vi "DriveSingleton.vi"(9 "Get/Set":enum16{"Get", "Set"}(ring), 11 "DriveBase.lvclass":refnum<class "DriveBase.lvclass">) -> (3 "DriveBase.lvclass 2":refnum<class "DriveBase.lvclass">)   [LabVIEW 2016, in "DriveBase.lvclass"]
uses:
  DriveBase.lvclass
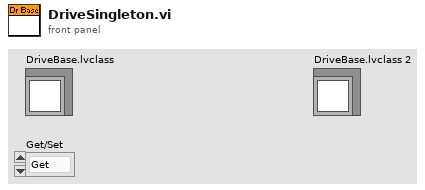
[diagram p1: front panel]
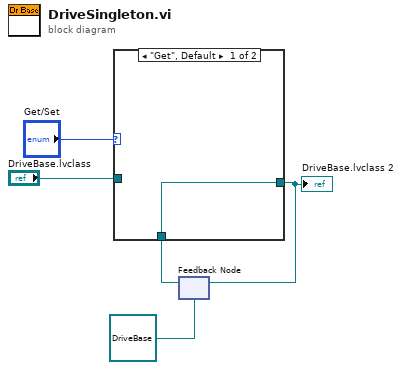
[diagram p0: block diagram]
diagram:
  n1 = feedback #1(refnum<class "DriveBase.lvclass"> refnum ("DriveBase.lvclass")) -> (w2:refnum<class "DriveBase.lvclass">)
  n2 = case shown="\"Get\", Default" "Get/Set" {
    tunnel: "DriveBase.lvclass" -> [_ w7]
    tunnel: [w6 w7] -> w1
    tunnel: w2 -> [w6 _]
    frame "Get", Default {
    }
    frame "Set" {
    }
  }
  "DriveBase.lvclass 2" <- w1
  n3 = feedback-in #1(w1) -> ()
